vi "Euler_ang_Sim2Table_conv(SubVI).vi"(11 "Euler Angles SIM[rad]":dbl[](array[numeric])) -> (3 "Euler Angles Table [deg]":dbl[](array[numeric]))   [LabVIEW 2011]
uses:
  <vilib>/Analysis/coordinate.llb/Euler Rotation Order.ctl
  <vilib>/Analysis/NI_AALPro.lvlib
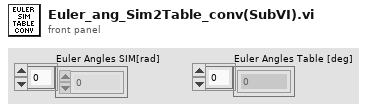
[diagram p1: front panel]
types:
  T1 = typedef "NI_AALPro.lvlib/Euler Rotation Order.ctl" = u16
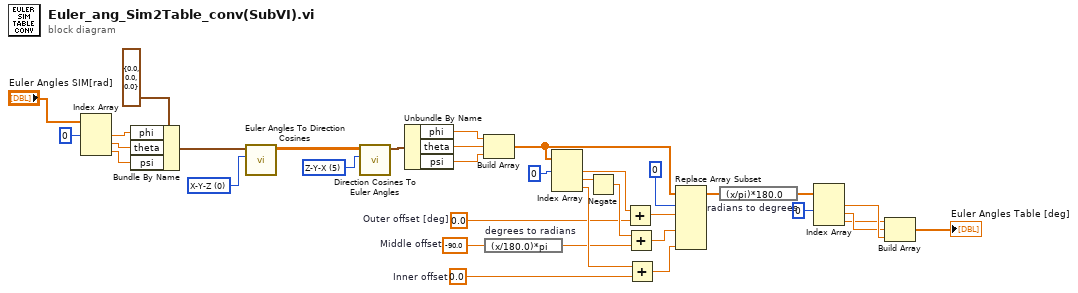
[diagram p0: block diagram]
diagram:
  w8 = 0.0  # Inner offset
  w23 = -90.0  # Middle offset
  w7 = 0.0  # Outer offset [deg]
  w11 = T1 5 items=["X-Y-Z", "X-Z-Y", "Y-X-Z", "Y-Z-X", "Z-X-Y", "Z-Y-X", "X-Y-X", "X-Z-X", "Y-X-Y", "Y-Z-Y", "Z-X-Z", "Z-Y-Z"] ("rotation order")
  w9 = T1 0 items=["X-Y-Z", "X-Z-Y", "Y-X-Z", "Y-Z-X", "Z-X-Y", "Z-Y-X", "X-Y-X", "X-Z-X", "Y-X-Y", "Y-Z-Y", "Z-X-Z", "Z-Y-Z"] ("rotation order")
  n1 = Index Array(array="Euler Angles SIM[rad]", index #1=0 ("index")) -> (element #1=w15:dbl, element #2=w16:dbl, element #3=w17:dbl)  [unwired: 2 in]
  n2 = Bundle By Name(cluster=cluster{"phi":dbl, "theta":dbl, "psi":dbl} {"phi"=0.0, "theta"=0.0, "psi"=0.0} ("Euler Angles"), "phi"=w15, "theta"=w16, "psi"=w17) -> (w13:cluster{"phi":dbl, "theta":dbl, "psi":dbl})
  n3 = call <vilib>:"Euler Angles To Direction Cosines.vi"("rotation order"=w9, "Euler Angles"=w13) -> ("Direction Cosines"=w10:dbl[][])  [unwired: 8 in, 1 out]
  n4 = call <vilib>:"Direction Cosines To Euler Angles.vi"("rotation order"=w11, "Direction Cosines"=w10) -> ("Euler Angles"=w18:cluster{"phi":dbl, "theta":dbl, "psi":dbl})  [unwired: 8 in, 1 out]
  n5 = Unbundle By Name(w18) -> ("phi"=w20:dbl, "theta"=w19:dbl, "psi"=w21:dbl)
  n6 = Build Array(w20, w19, w21) -> (w22:dbl[])
  n7 = expression code="(x/180.0)*pi" "degrees to radians"(w23) -> (w24:dbl)
  n8 = Index Array(array=w22, index #1=0 ("index")) -> (element #1=w5:dbl, element #2=w26:dbl, element #3=w33:dbl)  [unwired: 2 in]
  n9 = Negate(x=w26) -> (-x=w27:dbl)
  n10 = Add(x=w5, y=w7) -> (x+y=w2:dbl)
  n11 = Add(x=w27, y=w24) -> (x+y=w3:dbl)
  n12 = Add(x=w33, y=w8) -> (x+y=w4:dbl)
  n13 = Replace Array Subset(array=w22, new element #1=w2, index #1=0 ("index"), new element #2=w3, new element #3=w4) -> (w25:dbl[])  [unwired: 2 in]
  n14 = expression code="(x/pi)*180.0" "radians to degrees"(w25) -> (w28:dbl[])
  n15 = Index Array(array=w28, index #1=0 ("index")) -> (element #1=w32:dbl, element #2=w31:dbl, element #3=w30:dbl)  [unwired: 2 in]
  n16 = Build Array(w30, w31, w32) -> (→"Euler Angles Table [deg]":dbl[])
